vi "read.vi"(8 "error in":errorcluster, 9 "timeout in ms (-1)":i32=-1, 11 "stream publisher in":refnum<class "subscriber.lvclass">) -> (0 "error out":errorcluster, 1 "timed out?":bool, 2 "element":T1, 3 "stream publisher out":refnum<class "subscriber.lvclass">)   [LabVIEW 2013, in "data stream.lvlib" / "subscriber.lvclass"]
uses:
  subscriber.lvclass
  stream definition.ctl
  message definition.ctl
  subscriber.lvclass/subscriber.ctl
  data stream.lvlib
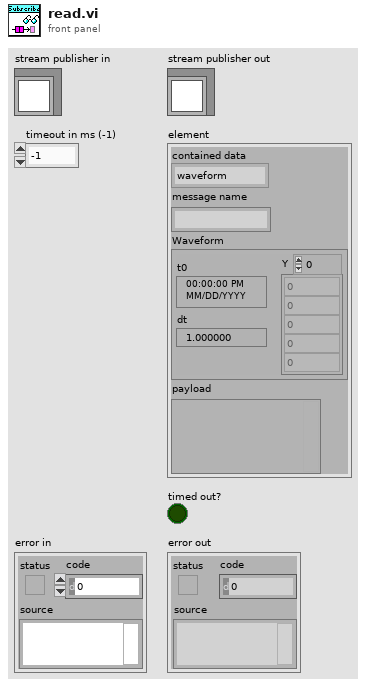
[diagram p1: front panel]
types:
  T1 = typedef "data stream.lvlib/stream definition.ctl" = cluster{"contained data":T2, "message name":string, "Waveform":waveform(dbl), "payload":variant}
  T2 = typedef "data stream.lvlib/message definition.ctl" = enum16{"waveform", "message"}
  T3 = typedef "data stream definition.ctl" = cluster{"contained data":T4, "message name":string, "Waveform":waveform(dbl), "payload":variant}
  T4 = typedef "data stream message type.ctl" = enum16{"waveform", "message"}
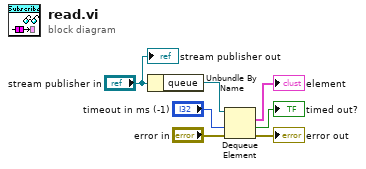
[diagram p0: block diagram]
diagram:
  n1 = Unbundle By Name("stream publisher in") -> ("queue"=w4:refnum<queue>)
  n2 = Dequeue Element(queue=w4, timeout in ms (-1)="timeout in ms (-1)", error in (no error)="error in") -> (element=→"element":T3, timed out?=→"timed out?":bool, error out=→"error out":errorcluster)  [unwired: 1 out]
  "stream publisher out" <- "stream publisher in"
